vi "MFC test.vi"() -> ()   [LabVIEW 2014]
uses:
  <vilib>/Instr/_visa.llb/VISA Configure Serial Port (Instr).vi
panel:
  in  "write buffer":string
  in  "Serial Settings":T1={"baud rate"=38400, "data bits"=8, "parity"=enum."None", "stop bits"=10, "flow control"=1} {"flow control" items=["None"=0, "XON/XOFF"=1, "RTS/CTS"=2, "DTR/DSR"=4]; "stop bits" items=["1.0"=10, "1.5"=15, "2.0"=20]; "data bits" min=5 max=8 step=1; "baud rate" items=["75"=75, "110"=110, "134"=134, "150"=150, "300"=300, "600"=600, "1200"=1200, "1800"=1800, "2400"=2400, "4800"=4800, "7200"=7200, "9600"=9600, "14400"=14400, "19200"=19200, "28800"=28800, "19200"=38400, "56000"=56000, "57600"=57600, "115200"=115200, "128000"=128000, "230400"=230400]}
  in  "VISA RS 485 Resource":refnum<visa-resource-name>="COM6"
  out "error out":errorcluster={"status"=TRUE, "code"=-1073807339, "source"="VISA Read in MFC test.vi"}
  in  "byte count":u32=64
  out "Serial Settings:Number of Bytes at Serial Port":u32
  out "Array":string[](array[string])
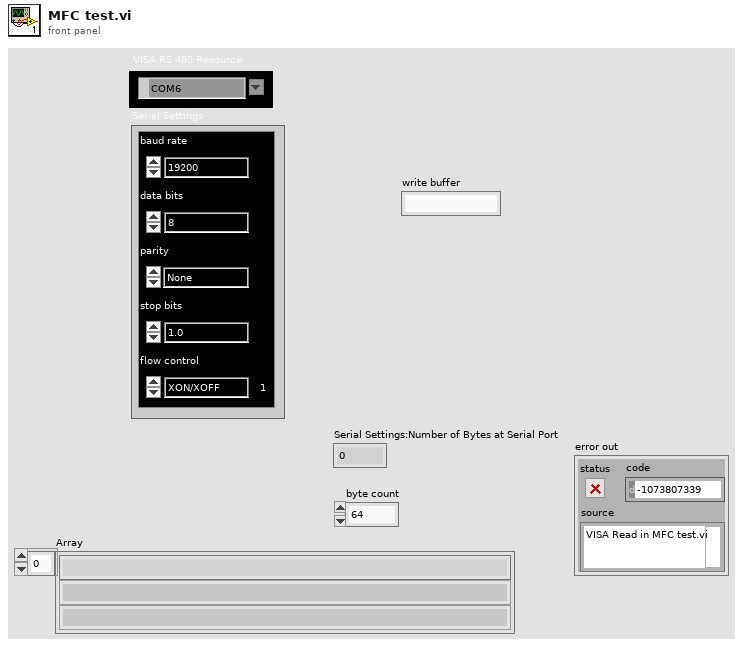
[diagram p1: front panel]
types:
  T1 = cluster{"baud rate":u32, "data bits":u16, "parity":enum16{"None", "Odd", "Even", "Mark", "Space"}, "stop bits":u16, "flow control":u16}
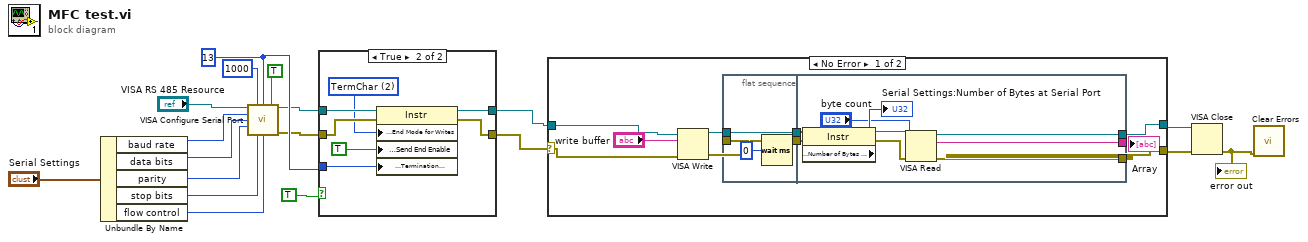
[diagram p0: block diagram]
diagram:
  w6 = u8 13 ("Termination Character")
  n1 = Unbundle By Name("Serial Settings") -> ("baud rate"=w13:u32, "data bits"=w12:u16, "parity"=w11:enum16{"None", "Odd", "Even", "Mark", "Space"}, "stop bits"=w10:u16, "flow control"=w9:u16)
  n2 = call-poly "VISA Configure Serial Port"("VISA resource name"="VISA RS 485 Resource", "timeout (10sec)"=u32 1000, "termination char\n(0xA = '\\n' = LF)"=w6, "Enable Termination\nChar (T)"=TRUE ("End Read on Termination Character?"), "baud rate (9600)"=w13, "data bits (8)"=w12, "parity (0:none)"=w11, "stop bits (10: 1 bit)"=w10, "flow control (0:none)"=w9) -> ("VISA resource name out"=w5:refnum<visa-resource-name>, "error out"=w4:errorcluster)  [unwired: 1 in, 4 out]
  n3 = case shown="True" TRUE ("End Write on Termination Character?") {
    tunnel: w5 -> [w19 w27]
    tunnel: w4 -> [w20 w26]
    tunnel: [w19 w25] -> w2
    tunnel: [w20 w24] -> w3
    tunnel: w6 -> [_ w22]
    frame False {
    }
    frame True {
      w23 = u16 2 items=["None", "LastBit", "TermChar", "Break"] ("Serial Settings:Serial End Mode for Writes")
      n4 = property class="Instr"(reference=w27, error in=w26, "Serial Settings:End Mode for Writes"=w23, "Message Based Settings:Send End Enable"=TRUE, "Message Based Settings:Termination Character"=w22) -> (reference out=w25:refnum<visa-resource-name>, error out=w24:errorcluster)
    }
  }
  n5 = case shown="No Error" w3 {
    selector: w3 -> [w35 w49]
    tunnel: w2 -> [w36 w50]
    tunnel: [w34 w49] -> w18
    tunnel: [w33 w50] -> w17
    frame No Error {
      n6 = VISA Write(VISA resource name=w36, write buffer="write buffer", error in (no error)=w35) -> (VISA resource name out=w30:refnum<visa-resource-name>, error out=w29:errorcluster)  [unwired: 1 out]
      n7 = flat-sequence {
        tunnel: w29 -> [w38]
        tunnel: w30 -> [w39]
        tunnel: [w39] -> w32
        tunnel: [w38] -> w31
        tunnel: [w44] -> w34
        tunnel: [w43] -> w33
        tunnel: [w42] -> _
        tunnel: w32 -> [w48]
        tunnel: w31 -> [w45]
        frame #0 {
          n8 = Wait (ms)(milliseconds to wait=u32 0) -> ()  [unwired: 1 out]
        }
        frame #1 {
          n9 = property class="Instr"(reference=w48, error in=w45) -> (reference out=w47:refnum<visa-resource-name>, error out=w46:errorcluster, "Serial Settings:Number of Bytes at Serial Port"=→"Serial Settings:Number of Bytes at Serial Port":u32)
          n10 = VISA Read(VISA resource name=w47, byte count="byte count", error in (no error)=w46) -> (VISA resource name out=w43:refnum<visa-resource-name>, read buffer=w42:string, error out=w44:errorcluster)  [unwired: 1 out]
        }
      }
    }
    frame Error {
    }
  }
  n11 = VISA Close(VISA resource name=w17, error in (no error)=w18) -> (error out=w16:errorcluster)
  "error out" <- w16
  n12 = call <vilib>:"Clear Errors.vi"("error in (no error)"=w16) -> ()  [unwired: 5 in, 2 out]
